vi "act 19.vi"() -> ()   [LabVIEW 2010]
uses:
  act/lv_07/lv_07.lvlib
panel:
  out "Te (en mois)":dbl
  in  "Cc":dbl
  in  "T":dbl
  in  "error in":errorcluster caption="err out"
  out "err out":errorcluster caption="err in"
  out "Qe":dbl
  in  "Pu":dbl
  in  "Qa":dbl
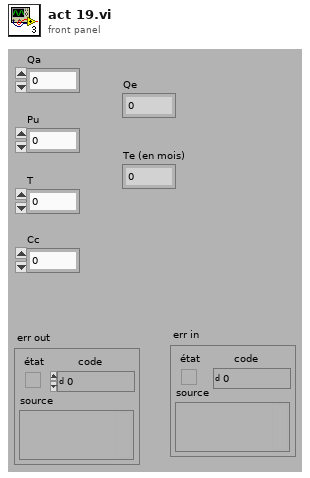
[diagram p1: front panel]
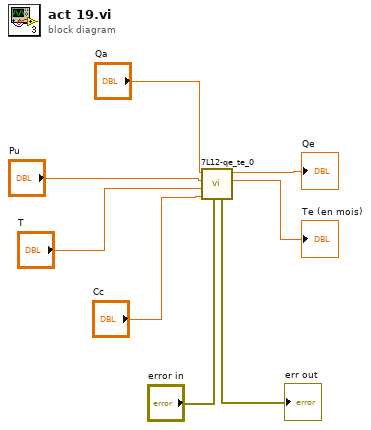
[diagram p0: block diagram]
diagram:
  n1 = call "7L12-qe_te_0.vi"("err in"="error in", "Cc"="Cc", "T"="T", "Pu"="Pu", "Qa"="Qa") -> ("Te (en mois)"=→"Te (en mois)":dbl, "Qe"=→"Qe":dbl, "error out"=→"err out":errorcluster)  [unwired: 4 in]
